vi "ListboxValueChange.vi"(8 "error in (no error)":errorcluster, 9 "OldVal":i32, 10 "NewVal":i32, 11 "ListBox in":refnum<vi>) -> (0 "error out":errorcluster)   [LabVIEW 2016, in "DisplayWindow.lvlib" / "DisplayWindow.lvclass"]
uses:
  DisplayWindow.lvclass
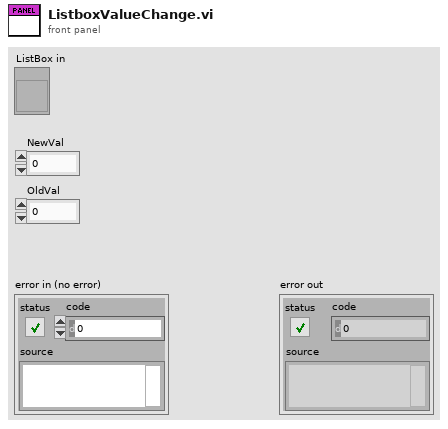
[diagram p1: front panel]
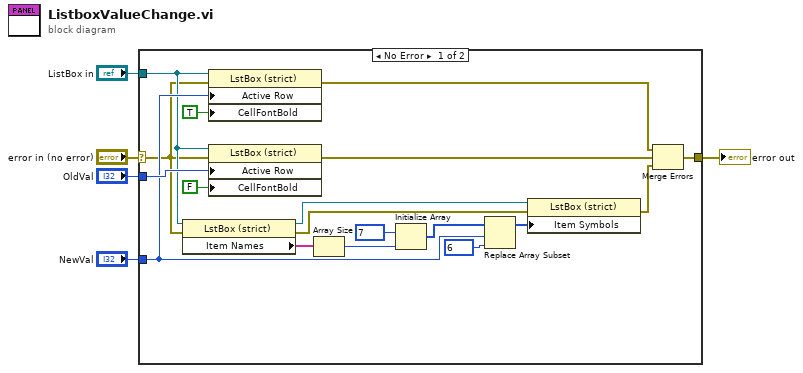
[diagram p0: block diagram]
diagram:
  n1 = case shown="No Error" "error in (no error)" {
    selector: "error in (no error)" -> [w9 w24]
    tunnel: "OldVal" -> [w21 _]
    tunnel: "ListBox in" -> [w13 _]
    tunnel: "NewVal" -> [w14 _]
    tunnel: [w8 w24] -> w1
    frame No Error {
      n2 = property on="Property Node" class="LstBox (strict)"(reference=w13, error in=w9) -> (reference out=w12:refnum<vi>, error out=w11:errorcluster, "Item Names"=w17:string[])
      n3 = property on="Property Node" class="LstBox (strict)"(reference=w13, error in=w9, "Active Row"=w14, "CellFontBold"=TRUE ("Active Row:Cell Font:Bold")) -> (error out=w7:errorcluster)  [unwired: 1 out]
      n4 = property on="Property Node" class="LstBox (strict)"(reference=w13, error in=w9, "Active Row"=w21, "CellFontBold"=FALSE ("Active Row:Cell Font:Bold")) -> (error out=w6:errorcluster)  [unwired: 1 out]
      n5 = Array Size(array=w17) -> (size(s)=w18:i32)
      n6 = Initialize Array(7, w18) -> (w15:i32[])
      n7 = Replace Array Subset(array=w15, new element=6, index=w14) -> (w16:i32[])
      n8 = property on="Property Node" class="LstBox (strict)"(reference=w12, error in=w11, "Item Symbols"=w16) -> (error out=w10:errorcluster)  [unwired: 1 out]
      n9 = Merge Errors(w7, w6, w10) -> (w8:errorcluster)
    }
    frame Error {
    }
  }
  "error out" <- w1
